vi "质控启动器.vi"(8 "error in (no error)":errorcluster, 9 "加标体积":sgl, 10 "流程控制":T1, 11 "Slave ID":T2) -> (0 "error out":errorcluster)   [LabVIEW 2016, in "质控单元V4.lvlib"]
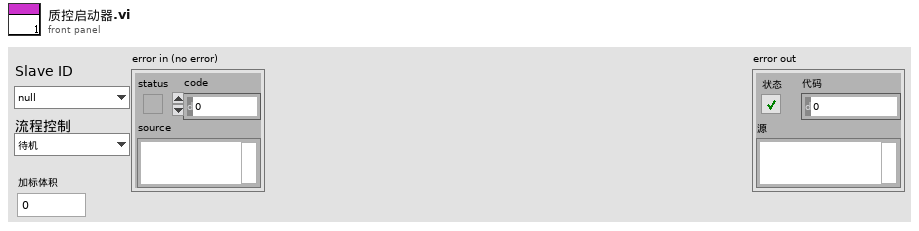
[diagram p1: front panel]
types:
  T1 = typedef "质控单元V4.lvlib/质控标准流程.ctl" = enum16{"待机", "启动进样流程", "启动加标流程", "启动排液流程", "启动水样润洗流程", "启动加标润洗流程", "停止流程", "启动搅拌流程", "停止搅拌流程"}
  T2 = typedef "质控单元V4.lvlib/质控slave id.ctl" = enum16{"null", "氨氮", "总磷", "总氮", "CODMn", "CODCr"}
  T3 = typedef "质控单元V4.lvlib/质控组合命令区.ctl" = enum16{"停止", "进水样", "排废液", "进空气（搅拌）", "定量（反转定量）"}
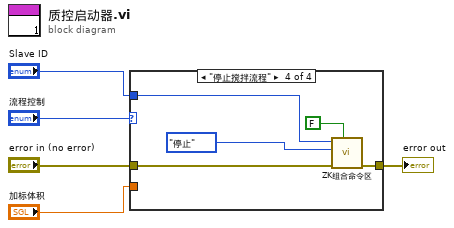
[diagram p0: block diagram]
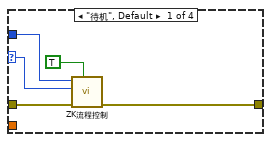
[diagram p2: hidden frame]
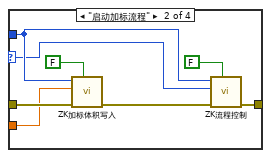
[diagram p3: hidden frame]
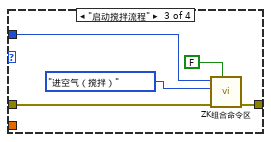
[diagram p4: hidden frame]
diagram:
  n1 = case shown="\"停止搅拌流程\"" "流程控制" {
    selector: "流程控制" -> [w8 w12 _ _]
    tunnel: "Slave ID" -> [w10 w13 w23 w28]
    tunnel: [w7 w14 w20 w25] -> w1
    tunnel: "error in (no error)" -> [w6 w17 w21 w26]
    tunnel: "加标体积" -> [_ w16 _ _]
    frame "待机", Default {
      n2 = call "ZK流程控制.vi"("是否启用通讯通知"=TRUE, "error in (no error)"=w6, "流程控制"=w8, "Slave ID"=w10) -> ("error out"=w7:errorcluster)  [unwired: 7 in]
    }
    frame "启动加标流程" {
      n3 = call "ZK加标体积写入.vi"("是否启用通讯通知"=FALSE, "error in (no error)"=w17, "加标体积"=w16, "Slave ID"=w13) -> ("error out"=w15:errorcluster)  [unwired: 7 in]
      n4 = call "ZK流程控制.vi"("是否启用通讯通知"=FALSE, "error in (no error)"=w15, "流程控制"=w12, "Slave ID"=w13) -> ("error out"=w14:errorcluster)  [unwired: 7 in]
    }
    frame "启动搅拌流程" {
      n5 = call "ZK组合命令区.vi"("是否启用通讯通知"=FALSE, "error in (no error)"=w21, "组合命令区"=质控组合命令区."进空气（搅拌）", "Slave ID"=w23) -> ("error out"=w20:errorcluster)  [unwired: 7 in]
    }
    frame "停止搅拌流程" {
      n6 = call "ZK组合命令区.vi"("是否启用通讯通知"=FALSE, "error in (no error)"=w26, "组合命令区"=质控组合命令区."停止", "Slave ID"=w28) -> ("error out"=w25:errorcluster)  [unwired: 7 in]
    }
  }
  "error out" <- w1
